vi "Plot Trajectory PtbyPt.vi"(7 "Reset? (F)":bool, 11 "State":T1) -> (3 "Telemetry":cluster{dbl[], dbl[]}[](graph))   [LabVIEW 2019]
uses:
  Typedef/Trajectory State.ctl
  Geometry/Typedef/Pose2d.ctl
  Geometry/Typedef/Translation2d.ctl
  Geometry/Typedef/Rotation2d.ctl
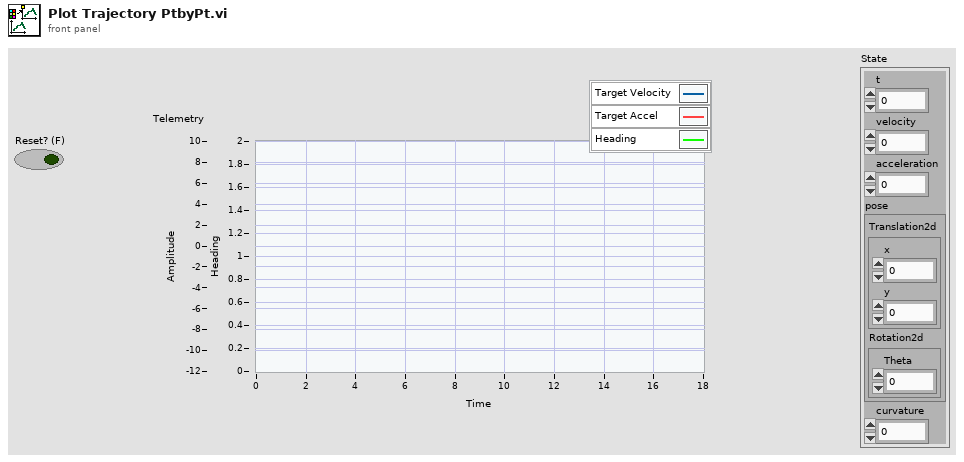
[diagram p1: front panel]
types:
  T1 = typedef "Trajectory State.ctl" = cluster{"t":dbl, "velocity":dbl, "acceleration":dbl, "pose":T2, "curvature":dbl}
  T2 = typedef "Pose2d.ctl" = cluster{"Translation2d":T3, "Rotation2d":T4}
  T3 = typedef "Translation2d.ctl" = cluster{"x":dbl, "y":dbl}
  T4 = typedef "Rotation2d.ctl" = cluster{"Theta":dbl}
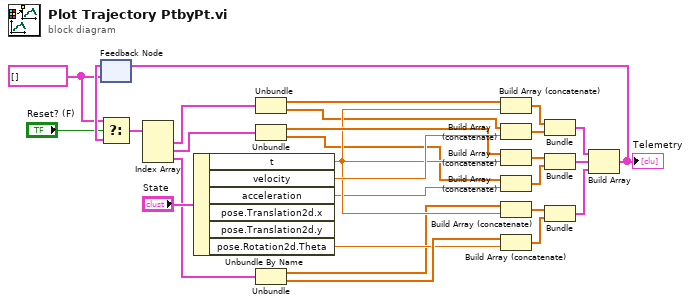
[diagram p0: block diagram]
diagram:
  w1 = cluster{dbl[], dbl[]}[] []
  n1 = feedback #1(w1) -> (w8:cluster{dbl[], dbl[]}[])
  n2 = Select(t=w1, s="Reset? (F)", f=w8) -> (s? t:f=w7:cluster{dbl[], dbl[]}[])
  n3 = Index Array(array=w7) -> (element #1=w27:cluster{dbl[], dbl[]}, element #2=w26:cluster{dbl[], dbl[]}, element #3=w25:cluster{dbl[], dbl[]})  [unwired: 3 in]
  n4 = Unbundle By Name("State") -> ("t"=w21:dbl, "velocity"=w24:dbl, "acceleration"=w20:dbl, "pose.Rotation2d.Theta"=w18:dbl)  [unwired: 2 out]
  n5 = Unbundle(w27) -> (w23:dbl[], w3:dbl[])
  n6 = Unbundle(w26) -> (w22:dbl[], w4:dbl[])
  n7 = Unbundle(w25) -> (w2:dbl[], w19:dbl[])
  n8 = Build Array (concatenate)(w23, w21) -> (w17:dbl[])
  n9 = Build Array (concatenate)(w3, w24) -> (w16:dbl[])
  n10 = Build Array (concatenate)(w22, w21) -> (w15:dbl[])
  n11 = Build Array (concatenate)(w4, w20) -> (w14:dbl[])
  n12 = Build Array (concatenate)(w2, w21) -> (w13:dbl[])
  n13 = Build Array (concatenate)(w19, w18) -> (w12:dbl[])
  n14 = Bundle(w17, w16) -> (w9:cluster{dbl[], dbl[]})  [unwired: 1 in]
  n15 = Bundle(w15, w14) -> (w10:cluster{dbl[], dbl[]})  [unwired: 1 in]
  n16 = Bundle(w13, w12) -> (w11:cluster{dbl[], dbl[]})  [unwired: 1 in]
  n17 = Build Array(w9, w10, w11) -> (w6:cluster{dbl[], dbl[]}[])
  "Telemetry" <- w6
  n18 = feedback-in #1(w6) -> ()
